vi "FixUnsetOptions.vi"(11 "Fileopts in":T1) -> (3 "Fileopts out":T1)   [LabVIEW 2012, in "configlib.lvlib"]
uses:
  configlib.lvlib
  File Options.ctl
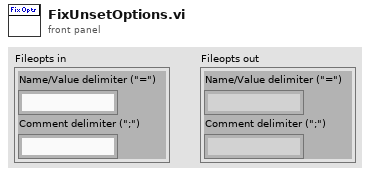
[diagram p1: front panel]
types:
  T1 = typedef "configlib.lvlib/File Options.ctl" = cluster{"Name/Value delimiter (\"=\")":string, "Comment delimiter (\";\")":string}
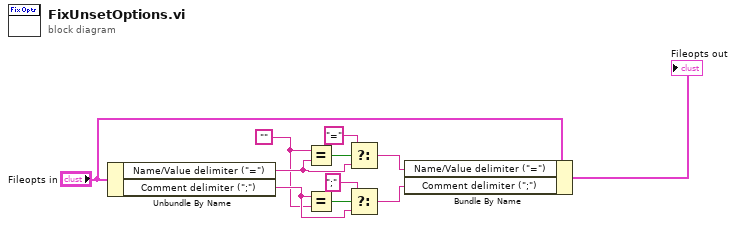
[diagram p0: block diagram]
diagram:
  w1 = ""
  n1 = Unbundle By Name("Fileopts in") -> ("Name/Value delimiter (\"=\")"=w4:string, "Comment delimiter (\";\")"=w5:string)
  n2 = Equal?(x=w1, y=w4) -> (x = y?=w2:bool)
  n3 = Equal?(x=w5, y=w1) -> (x = y?=w3:bool)
  n4 = Select(t="=", s=w2, f=w4) -> (s? t:f=w10:string)
  n5 = Select(t=";", s=w3, f=w5) -> (s? t:f=w9:string)
  n6 = Bundle By Name(cluster="Fileopts in", "Name/Value delimiter (\"=\")"=w10, "Comment delimiter (\";\")"=w9) -> (→"Fileopts out":T1)
